vi "roboRIO v1.0 Reset Encoder.vi"(8 "error in (no error)":errorcluster, 10 "Channel":T1, 11 "myRIO Ref In":T2) -> (0 "error out":errorcluster, 3 "myRIO Ref Out":T2)   [LabVIEW 2021]
uses:
  <vilib>/myRIO/Common/Instrument Driver Framework/Utilities/typedefs/myRIO v1.0 Reference.ctl
  <vilib>/myRIO/Common/Instrument Driver Framework/Utilities/typedefs/Generic FPGA Reference.ctl
  <vilib>/myRIO/Common/Instrument Driver Framework/myRIO v1.0/Encoder/typedefs/Encoder Channels Enum.ctl
  <vilib>/myRIO/Common/Instrument Driver Framework/roboRIO v1.0/Encoder/typedefs/roboRIO Encoder Channels FPGA Reference.ctl
  <vilib>/rvi/errors/niLvFpgaAdjustHostInterfaceError.vi
  <vilib>/rvi/interface/nirviReadWriteControl/nirviReadWriteControl.xnode
  <vilib>/rvi/interface/Simulation/niFpgaSimulationCallBeginRW.vi
  NiFpgaLv.dll
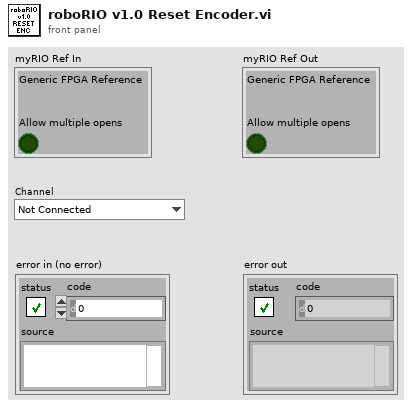
[diagram p1: front panel]
types:
  T1 = typedef "Encoder Channels Enum.ctl" = enum16{"Not Connected", "C/ENC0", "C/ENC1", "A/ENC", "A/ENC0", "A/ENC1", "A/ENC2", "A/ENC3", "A/ENC4", "A/ENC5", "A/ENC6", "A/ENC7", "A/ENC8", "A/ENC9", "B/ENC", "B/ENC0", "B/ENC1", "B/ENC2", "B/ENC3", "B/ENC4", "B/ENC5", "B/ENC6", "B/ENC7", "B/ENC8", "B/ENC9", "DIO/ENC0", "DIO/ENC1", "DIO/ENC2", "DIO/ENC3", "DIO/ENC4"}
  T2 = typedef "myRIO v1.0 Reference.ctl" = cluster{"Generic FPGA Reference":T3, "Allow multiple opens":bool}
  T3 = typedef "Generic FPGA Reference.ctl" = refnum<k20>
  T4 = typedef "roboRIO Encoder Channels FPGA Reference.ctl" = refnum<k20>
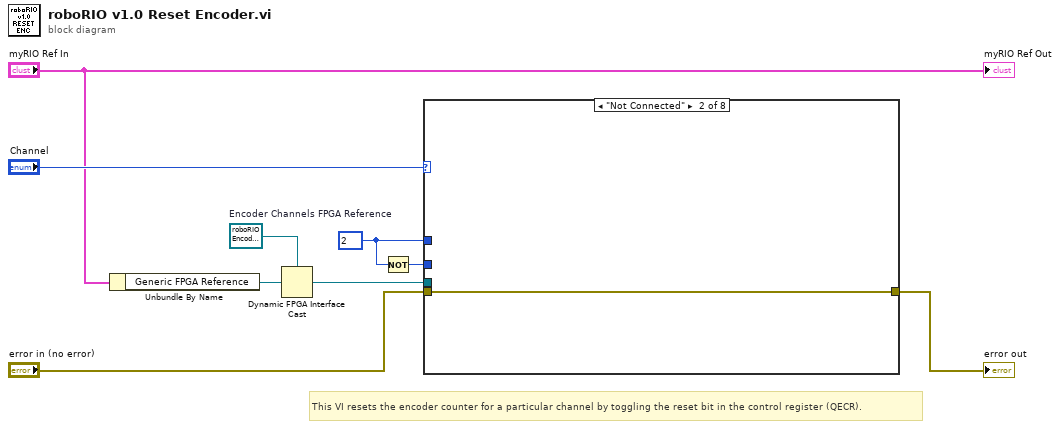
[diagram p0: block diagram]
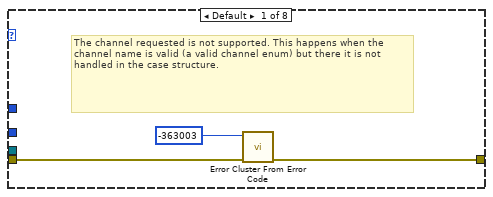
[diagram p2: hidden frame]
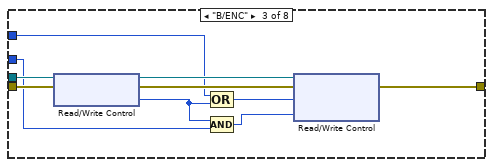
[diagram p3: hidden frame]
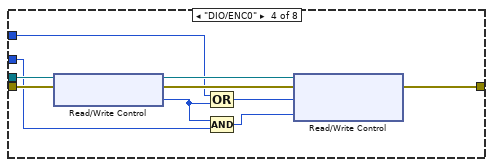
[diagram p4: hidden frame]
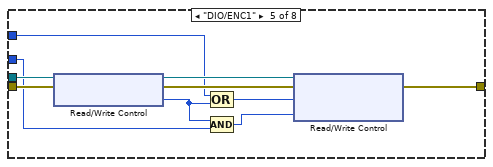
[diagram p5: hidden frame]
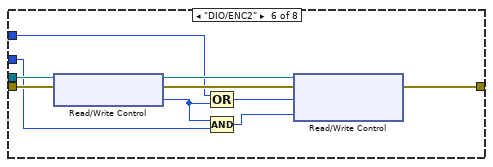
[diagram p6: hidden frame]
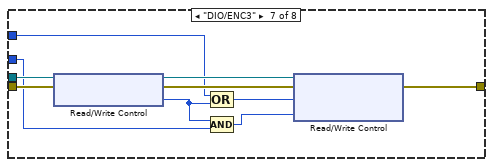
[diagram p7: hidden frame]
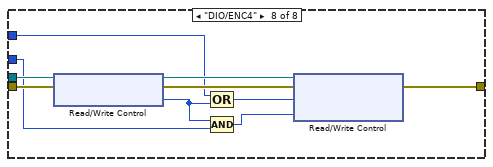
[diagram p8: hidden frame]
diagram:
  w4 = u8 2
  w9 = T4 refnum  # Encoder Channels FPGA Reference
  # "This VI resets the encoder counter for a particular channel by toggling the reset bit in the control register (QECR)."
  n1 = Unbundle By Name("myRIO Ref In") -> ("Generic FPGA Reference"=w2:T3)
  n2 = Dynamic FPGA Interface Cast(Session In=w9, Type=w2) -> (Session Out=w8:T4)
  n3 = Not(x=w4) -> (.not. x?=w3:u8)
  n4 = case shown="\"Not Connected\"" "Channel" {
    tunnel: "error in (no error)" -> [w10 w13 w19 w29 w39 w49 w59 w69]
    tunnel: [w11 w13 w23 w33 w43 w53 w63 w73] -> w5
    tunnel: w8 -> [_ _ w20 w30 w40 w50 w60 w70]
    tunnel: w4 -> [_ _ w18 w28 w38 w48 w58 w68]
    tunnel: w3 -> [_ _ w15 w25 w35 w45 w55 w65]
    frame Default {
      # "The channel requested is not supported. This happens when the channel name is valid (a valid channel enum) but there it is not handled in the case structure."
      n5 = call <vilib>:"Error Cluster From Error Code.vi"("error in (no error)"=w10, "error code (0)"=-363003) -> ("error out"=w11:errorcluster)  [unwired: 7 in]
    }
    frame "Not Connected" {
    }
    frame "B/ENC" {
      n6 = xnode "Read/Write Control"("FPGA VI Reference In"=w20, "error in"=w19) -> ("FPGA VI Reference Out"=w21:T4, "error out"=w22:errorcluster, "ENC.B.CNFG"=w14:u8)
      n7 = Compound Arithmetic op=OR(w18, w14) -> (w17:u8)
      n8 = Compound Arithmetic op=AND(w14, w15) -> (w16:u8)
      n9 = xnode "Read/Write Control"("FPGA VI Reference In"=w21, "error in"=w22, "ENC.B.CNFG"=w17, "ENC.B.CNFG"=w16) -> ("error out"=w23:errorcluster)  [unwired: 1 out]
    }
    frame "DIO/ENC0" {
      n10 = xnode "Read/Write Control"("FPGA VI Reference In"=w30, "error in"=w29) -> ("FPGA VI Reference Out"=w31:T4, "error out"=w32:errorcluster, "ENC.DIO_0.CNFG"=w24:u8)
      n11 = Compound Arithmetic op=OR(w28, w24) -> (w27:u8)
      n12 = Compound Arithmetic op=AND(w24, w25) -> (w26:u8)
      n13 = xnode "Read/Write Control"("FPGA VI Reference In"=w31, "error in"=w32, "ENC.DIO_0.CNFG"=w27, "ENC.DIO_0.CNFG"=w26) -> ("error out"=w33:errorcluster)  [unwired: 1 out]
    }
    frame "DIO/ENC1" {
      n14 = xnode "Read/Write Control"("FPGA VI Reference In"=w40, "error in"=w39) -> ("FPGA VI Reference Out"=w41:T4, "error out"=w42:errorcluster, "ENC.DIO_1.CNFG"=w34:u8)
      n15 = Compound Arithmetic op=OR(w38, w34) -> (w37:u8)
      n16 = Compound Arithmetic op=AND(w34, w35) -> (w36:u8)
      n17 = xnode "Read/Write Control"("FPGA VI Reference In"=w41, "error in"=w42, "ENC.DIO_1.CNFG"=w37, "ENC.DIO_1.CNFG"=w36) -> ("error out"=w43:errorcluster)  [unwired: 1 out]
    }
    frame "DIO/ENC2" {
      n18 = xnode "Read/Write Control"("FPGA VI Reference In"=w50, "error in"=w49) -> ("FPGA VI Reference Out"=w51:T4, "error out"=w52:errorcluster, "ENC.DIO_2.CNFG"=w44:u8)
      n19 = Compound Arithmetic op=OR(w48, w44) -> (w47:u8)
      n20 = Compound Arithmetic op=AND(w44, w45) -> (w46:u8)
      n21 = xnode "Read/Write Control"("FPGA VI Reference In"=w51, "error in"=w52, "ENC.DIO_2.CNFG"=w47, "ENC.DIO_2.CNFG"=w46) -> ("error out"=w53:errorcluster)  [unwired: 1 out]
    }
    frame "DIO/ENC3" {
      n22 = xnode "Read/Write Control"("FPGA VI Reference In"=w60, "error in"=w59) -> ("FPGA VI Reference Out"=w61:T4, "error out"=w62:errorcluster, "ENC.DIO_3.CNFG"=w54:u8)
      n23 = Compound Arithmetic op=OR(w58, w54) -> (w57:u8)
      n24 = Compound Arithmetic op=AND(w54, w55) -> (w56:u8)
      n25 = xnode "Read/Write Control"("FPGA VI Reference In"=w61, "error in"=w62, "ENC.DIO_3.CNFG"=w57, "ENC.DIO_3.CNFG"=w56) -> ("error out"=w63:errorcluster)  [unwired: 1 out]
    }
    frame "DIO/ENC4" {
      n26 = xnode "Read/Write Control"("FPGA VI Reference In"=w70, "error in"=w69) -> ("FPGA VI Reference Out"=w71:T4, "error out"=w72:errorcluster, "ENC.DIO_4.CNFG"=w64:u8)
      n27 = Compound Arithmetic op=OR(w68, w64) -> (w67:u8)
      n28 = Compound Arithmetic op=AND(w64, w65) -> (w66:u8)
      n29 = xnode "Read/Write Control"("FPGA VI Reference In"=w71, "error in"=w72, "ENC.DIO_4.CNFG"=w67, "ENC.DIO_4.CNFG"=w66) -> ("error out"=w73:errorcluster)  [unwired: 1 out]
    }
  }
  "error out" <- w5
  "myRIO Ref Out" <- "myRIO Ref In"
